vi "ritter sample 2.vi"() -> ()   [LabVIEW 2020]
doc: "Each half second this this program reads the current flow and accumulated volume. It calculates the average flow over the last 2 minutes and displays all data in a graph. On start-up it displays information on the gasflowmeter and allows to reset the accumulated volume to 0."
uses:
  <vilib>/Analysis/baseanly.llb/Mean (DBL).vi
  <vilib>/Analysis/NI_AALBase.lvlib
panel:
  in  "VISA in":refnum<visa-resource-name>="COM10"
  out "chart":T1(graph)
  in  "reset?":bool
  out "profile":string
  out "volume (l)":dbl
  in  "stop":bool
  out "flow (l/h)":dbl format="%.2f"
  out "flow (l/h) avg":dbl format="%.2f"
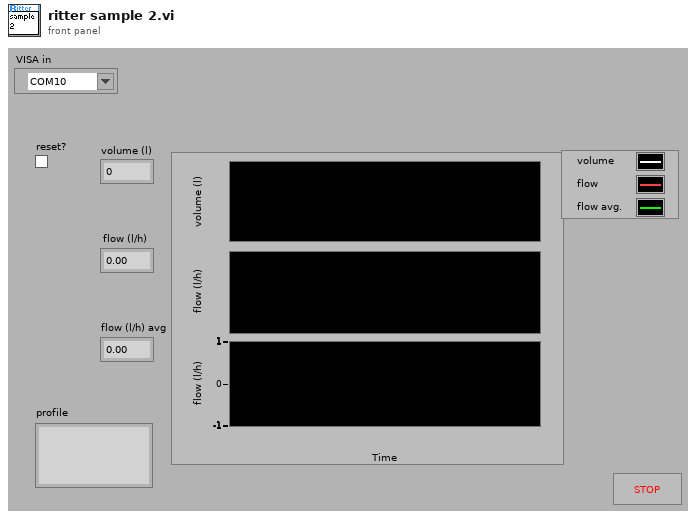
[diagram p1: front panel]
types:
  T1 = cluster{"volume (l)":dbl, "flow (l/h)":dbl, "mean":dbl}
  T2 = cluster{"volume (cuft)":dbl, "flow (cuft/hr)":dbl, "mean":dbl}
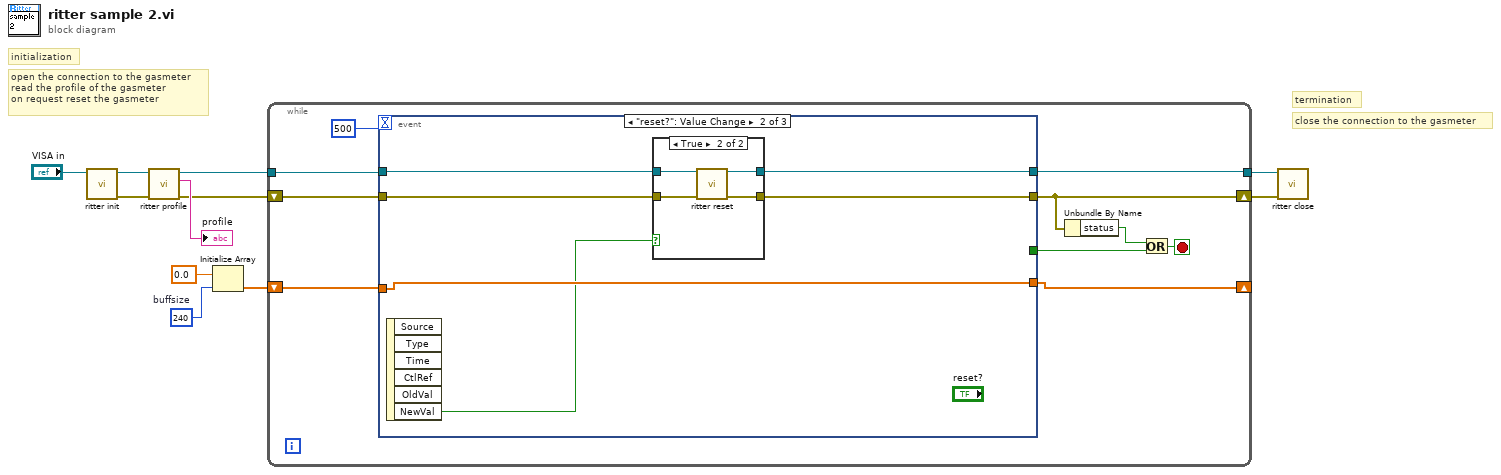
[diagram p0: block diagram]
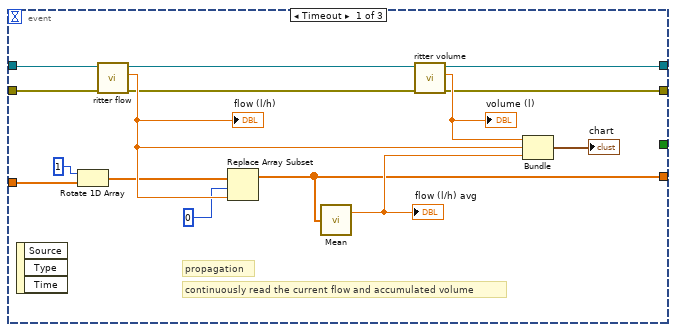
[diagram p2: hidden frame]
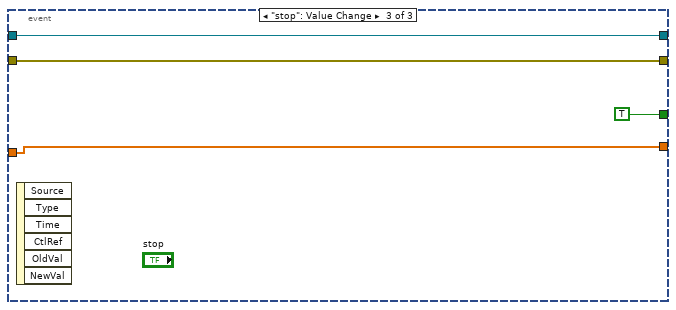
[diagram p4: hidden frame]
diagram:
  w11 = 240  # buffsize
  # "close the connection to the gasmeter"
  # "initialization"
  # "open the connection to the gasmeter\nread the profile of the gasmeter\non request reset the gasmeter"
  # "termination"
  n1 = call "ritter init.vi"("VISA in"="VISA in") -> ("error out"=w8:errorcluster, "VISA out"=w7:refnum<visa-resource-name>)  [unwired: 9 in]
  n2 = call "ritter profile.vi"("error in (no error)"=w8, "VISA in"=w7) -> ("error out"=w1:errorcluster, "profile"=→"profile":string, "VISA out"=w2:refnum<visa-resource-name>)  [unwired: 7 in]
  n3 = Initialize Array(0.0, w11) -> (w9:dbl[])
  n4 = while {
    shift-left: w9 -> [w17]
    shift-right: [w14] -> _
    tunnel: w2 -> [w18]
    tunnel: [w15] -> w5
    shift-right: [w16] -> w4
    shift-left: w1 -> [w19]
    stop <- w20 stop-if-true
    n5 = event shown="[1] \"reset?\": Value Change" {
      selector: _ -> [_ _ _]
      dyn-events: _ -> [_ _ _]
      timeout: u32 500 ("millisecond multiple") -> [_ _ _]
      tunnel: w19 -> [w29 w41 w49]
      tunnel: w18 -> [w28 w42 w50]
      tunnel: w17 -> [w26 w38 w51]
      tunnel: [w24 w40 w49] -> w16
      tunnel: [w23 w39 w50] -> w15
      tunnel: [w22 w38 w51] -> w14
      tunnel: [_ _ TRUE] -> w12
      event Timeout {
        # "propagation"
        # "continuously read the current flow and accumulated volume"
        n6 = event-data() -> ()  [unwired: 1 in, 3 out]
        n7 = Rotate 1D Array(1:w26, 2:1) -> (0:w30:dbl[])
        n8 = call "ritter flow.vi"("error in (no error)"=w29, "VISA in"=w28) -> ("error out"=w32:errorcluster, "flow (cuft/hr)"=w34:dbl, "VISA out"=w31:refnum<visa-resource-name>)  [unwired: 6 in, 1 out]
        "flow (l/h)" <- w34
        n9 = Replace Array Subset(array=w30, new element=w34, index=0) -> (w22:dbl[])
        n10 = call-poly <vilib>:"Mean.vi"("X"=w22) -> ("mean"=w35:dbl)  [unwired: 1 out]
        "flow (l/h) avg" <- w35
        n11 = call "ritter volume.vi"("error in (no error)"=w32, "VISA in"=w31) -> ("error out"=w24:errorcluster, "volume (cuft)"=w33:dbl, "VISA out"=w23:refnum<visa-resource-name>)  [unwired: 6 in, 1 out]
        "volume (l)" <- w33
        n12 = Bundle("volume (cuft)"=w33, "flow (cuft/hr)"=w34, "mean"=w35) -> (→"chart":T2)  [unwired: 1 in]
      }
      event "reset?": Value Change {
        n13 = event-data() -> ("NewVal"=w37:bool)  [unwired: 1 in, 5 out]
        n14 = case shown="True" w37 {
          tunnel: w42 -> [w43 w48]
          tunnel: w41 -> [w44 w47]
          tunnel: [w44 w46] -> w40
          tunnel: [w43 w45] -> w39
          frame False {
          }
          frame True {
            n15 = call "ritter reset.vi"("error in (no error)"=w47, "VISA in"=w48) -> ("error out"=w46:errorcluster, "VISA out"=w45:refnum<visa-resource-name>)  [unwired: 8 in]
          }
        }
      }
      event "stop": Value Change {
        n16 = event-data() -> ()  [unwired: 1 in, 6 out]
      }
    }
    n17 = Unbundle By Name(w16) -> ("status"=w21:bool)
    n18 = Or(x=w21, y=w12) -> (x .or. y?=w20:bool)
  }
  n19 = call "ritter close.vi"("error in (no error)"=w4, "VISA in"=w5) -> ()  [unwired: 9 in, 1 out]
